vi "Dialog Box.vi"(8 "error in (no error)":errorcluster, 11 "Dialog in":refnum<class "Dialog.lvclass">) -> (0 "error out":errorcluster, 1 "timed out?":bool, 2 "Selection":string, 3 "Dialog out":refnum<class "Dialog.lvclass">)   [LabVIEW 2012, in "Dialog.lvlib" / "Dialog.lvclass"]
doc: "This VI contains the code for the dialog box.\nOverride this VI to provide more functionality or to create your own application-specific dialog box."
uses:
  Dialog.lvclass
  Fading/_Fade In(I32).vi
panel:
  out "String":string
  in  "OK Button":bool
  # "Message"
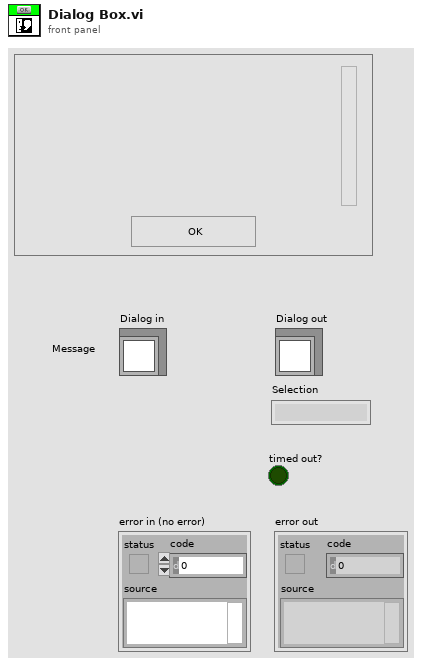
[diagram p1: front panel]
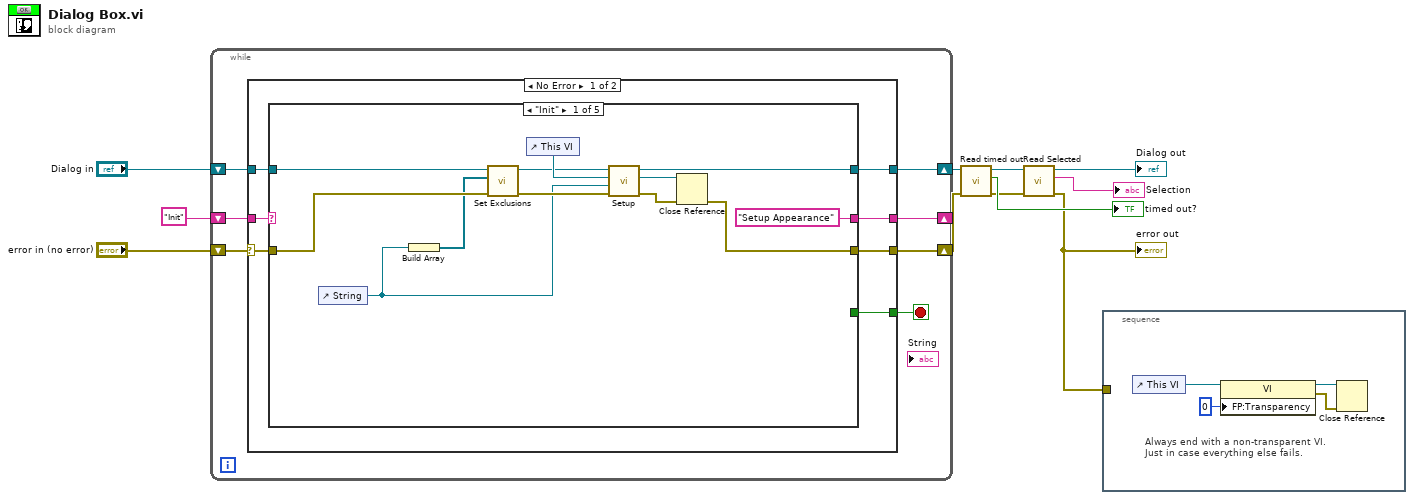
[diagram p0: block diagram]
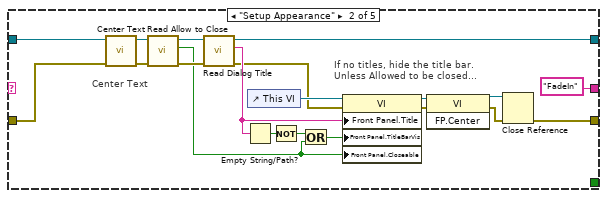
[diagram p2: hidden frame]
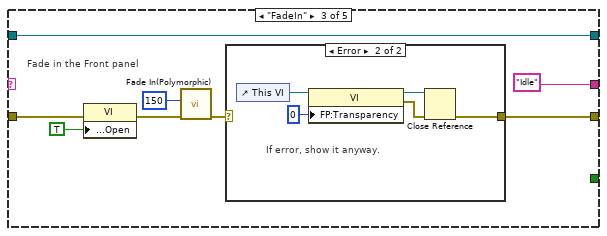
[diagram p3: hidden frame]
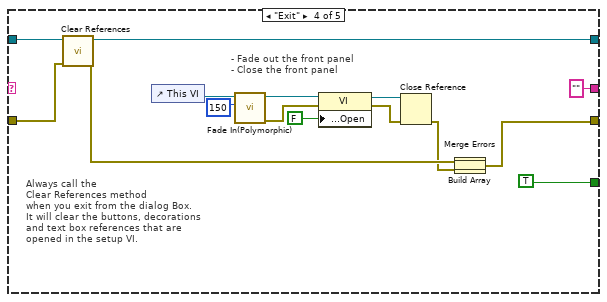
[diagram p5: hidden frame]
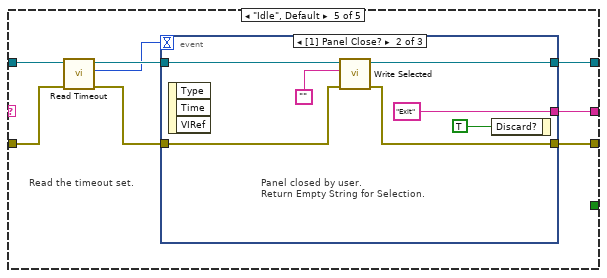
[diagram p6: hidden frame]
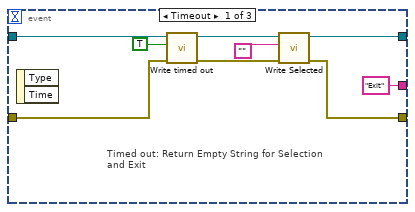
[diagram p7: hidden frame]
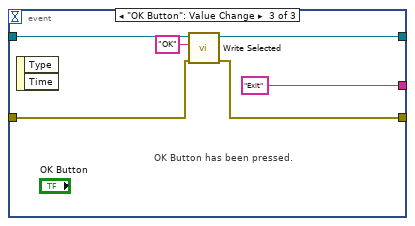
[diagram p8: hidden frame]
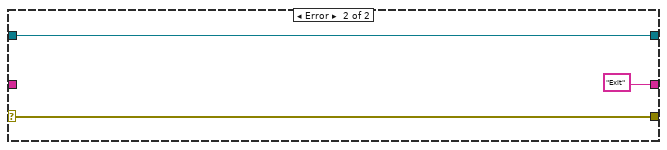
[diagram p9: hidden frame]
diagram:
  n1 = while {
    shift-right: [w14] -> _
    shift-left: "Init" -> [w15]
    shift-right: [w18] -> w4
    shift-left: "Dialog in" -> [w17]
    shift-right: [w16] -> w3
    shift-left: "error in (no error)" -> [w12]
    stop <- w13 stop-if-true
    n2 = case shown="No Error" w12 {
      selector: w12 -> [w19 w120]
      tunnel: [w25 w118] -> w18
      tunnel: w17 -> [w24 w118]
      tunnel: [w23 w120] -> w16
      tunnel: w15 -> [w22 _]
      tunnel: [w21 "Exit"] -> w14
      tunnel: [w20 _] -> w13
      frame No Error {
        n3 = case shown="\"Init\"" w22 {
          tunnel: [w35 w48 w65 w77 w95] -> w25
          tunnel: w24 -> [w31 w39 w65 w78 w92]
          tunnel: [w32 w49 w61 w73 w94] -> w23
          tunnel: w19 -> [w28 w38 w60 w76 w89]
          tunnel: ["Setup Appearance" "FadeIn" "Idle" "" w93] -> w21
          tunnel: [_ _ _ TRUE _] -> w20
          frame "Init" {
            n4 = control-ref of="String"() -> (w27:refnum<vi>)
            n5 = Build Array(w27) -> (w26:refnum<vi>[])
            n6 = call-dynamic "Set Exclusions.vi"("error in (no error)"=w28, "Exclusions"=w26, "Dialog in"=w31) -> ("error out"=w29:errorcluster, "Dialog out"=w30:refnum<class "Dialog.lvclass">)  [unwired: 7 out]
            n7 = control-ref of="This VI"() -> (w36:refnum<vi>)
            n8 = call-dynamic "Setup.vi"("error in (no error)"=w29, "Str Refnum"=w27, "VI Reference"=w36, "Dialog in"=w30) -> ("error out"=w33:errorcluster, "VI reference (dup)"=w34:refnum<vi>, "Dialog out"=w35:refnum<class "Dialog.lvclass">)  [unwired: 5 out]
            n9 = Close Reference(reference=w34, error in (no error)=w33) -> (error out=w32:errorcluster)
          }
          frame "Setup Appearance" {
            # "Center Text"
            # "If no titles, hide the title bar.\nUnless Allowed to be closed..."
            n10 = call-dynamic "Center Text.vi"("error in (no error)"=w38, "Dialog in"=w39) -> ("error out"=w44:errorcluster, "Dialog out"=w46:refnum<class "Dialog.lvclass">)  [unwired: 1 in, 7 out]
            n11 = call-dynamic "Read Allow to Close.vi"("error in (no error)"=w44, "Dialog.lvclass in"=w46) -> ("error out"=w43:errorcluster, "Allow to close?"=w40:bool, "Dialog.lvclass out"=w45:refnum<class "Dialog.lvclass">)  [unwired: 7 out]
            n12 = call-dynamic "Read Dialog Title.vi"("error in (no error)"=w43, "Dialog in"=w45) -> ("error out"=w47:errorcluster, "Dialog Title"=w52:string, "Dialog out"=w48:refnum<class "Dialog.lvclass">)  [unwired: 7 out]
            n13 = Empty String/Path?(string/path=w52) -> (empty?=w55:bool)
            n14 = control-ref of="This VI"() -> (w56:refnum<vi>)
            n15 = Not(x=w55) -> (.not. x?=w42:bool)
            n16 = Or(x=w42, y=w40) -> (x .or. y?=w41:bool)
            n17 = property class="VI"(reference=w56, error in=w47, "Front Panel.Title"=w52, "Front Panel.TitleBarVis"=w41, "Front Panel.Closeable"=w40) -> (reference out=w54:refnum<vi>, error out=w53:errorcluster)
            n18 = invoke class="VI" method="FP.Center"(reference=w54, error in=w53) -> (reference out=w51:refnum<vi>, error out=w50:errorcluster)  [unwired: 1 in, 1 out]
            n19 = Close Reference(reference=w51, error in (no error)=w50) -> (error out=w49:errorcluster)
          }
          frame "FadeIn" {
            # "Fade in the Front panel"
            n20 = property class="VI"(error in=w60, "Front Panel.Open"=TRUE ("Front Panel Window:Open")) -> (error out=w59:errorcluster)  [unwired: 1 in, 1 out]
            n21 = call-poly "Fade In(Polymorphic).vi"("error in"=w59, "Fade time (ms)"=150) -> ("error out"=w62:errorcluster)  [unwired: 2 in, 7 out]
            n22 = case shown="Error" w62 {
              selector: w62 -> [w66 _]
              tunnel: [w66 w67] -> w61
              frame No Error {
              }
              frame Error {
                # "If error, show it anyway."
                n23 = control-ref of="This VI"() -> (w69:refnum<vi>)
                n24 = property class="VI"(reference=w69, "FP:Transparency"=u8 0 ("Front Panel Window:Transparency")) -> (reference out=w70:refnum<vi>, error out=w71:errorcluster)  [unwired: 1 in]
                n25 = Close Reference(reference=w70, error in (no error)=w71) -> (error out=w67:errorcluster)
              }
            }
          }
          frame "Exit" {
            # "Always call the\nClear References method\nwhen you exit from the dialog Box.\nIt will clear the buttons, decorations\nand text box references that are \nopened in the setup VI."
            # "- Fade out the front panel\n- Close the front panel"
            n26 = call-dynamic "Clear References.vi"("error in (no error)"=w76, "Dialog in"=w78) -> ("error out"=w75:errorcluster, "Dialog out"=w77:refnum<class "Dialog.lvclass">)  [unwired: 8 out]
            n27 = control-ref of="This VI"() -> (w84:refnum<vi>)
            n28 = call-poly "Fade In(Polymorphic).vi"("Fade time (ms)"=150, "VI Reference (calling VI)"=w84) -> ("error out"=w82:errorcluster, "dup VI Reference"=w83:refnum<vi>)  [unwired: 2 in, 6 out]
            n29 = property class="VI"(reference=w83, error in=w82, "Front Panel.Open"=FALSE ("Front Panel Window:Open")) -> (reference out=w80:refnum<vi>, error out=w79:errorcluster)
            n30 = Close Reference(reference=w80, error in (no error)=w79) -> (error out=w74:errorcluster)
            n31 = Build Array(w75, w74) -> (w72:errorcluster[])
            n32 = Merge Errors(w72) -> (w73:errorcluster)
          }
          frame "Idle", Default {
            # "Read the timeout set."
            n33 = call-dynamic "Read Timeout.vi"("error in (no error)"=w89, "Dialog.lvclass in"=w92) -> ("error out"=w88:errorcluster, "Timeout"=w90:i32, "Dialog.lvclass out"=w91:refnum<class "Dialog.lvclass">)  [unwired: 7 out]
            n34 = event shown="[1] Panel Close?" {
              selector: _ -> [_ _ _]
              dyn-events: _ -> [_ _ _]
              timeout: w90 -> [_ _ _]
              tunnel: [w97 w107 w115] -> w95
              tunnel: w91 -> [w103 w108 w116]
              tunnel: [w98 w105 w112] -> w94
              tunnel: w88 -> [w101 w106 w113]
              tunnel: ["Exit" "Exit" "Exit"] -> w93
              event Timeout {
                # "Timed out: Return Empty String for Selection\nand Exit"
                n35 = event-data() -> ()  [unwired: 3 out]
                n36 = call-dynamic "Write timed out.vi"("error in (no error)"=w101, "timed out?"=TRUE, "Dialog.lvclass in"=w103) -> ("error out"=w99:errorcluster, "Dialog.lvclass out"=w100:refnum<class "Dialog.lvclass">)  [unwired: 7 out]
                n37 = call-dynamic "Write Selected.vi"("error in (no error)"=w99, "Selected"="", "Dialog.lvclass in"=w100) -> ("error out"=w98:errorcluster, "Dialog.lvclass out"=w97:refnum<class "Dialog.lvclass">)  [unwired: 7 out]
              }
              event Panel Close? {
                # "Panel closed by user.\nReturn Empty String for Selection."
                n38 = event-data() -> ()  [unwired: 4 out]
                n39 = call-dynamic "Write Selected.vi"("error in (no error)"=w106, "Selected"="", "Dialog.lvclass in"=w108) -> ("error out"=w105:errorcluster, "Dialog.lvclass out"=w107:refnum<class "Dialog.lvclass">)  [unwired: 7 out]
                n40 = event-data("Discard?"=TRUE) -> ()  [unwired: 1 in, 1 out]
              }
              event "OK Button": Value Change {
                # "OK Button has been pressed."
                n41 = event-data() -> ()  [unwired: 3 out]
                n42 = call-dynamic "Write Selected.vi"("error in (no error)"=w113, "Selected"="OK", "Dialog.lvclass in"=w116) -> ("error out"=w112:errorcluster, "Dialog.lvclass out"=w115:refnum<class "Dialog.lvclass">)  [unwired: 7 out]
              }
            }
          }
        }
      }
      frame Error {
      }
    }
  }
  n43 = call-dynamic "Read timed out.vi"("error in (no error)"=w3, "Dialog.lvclass in"=w4) -> ("error out"=w1:errorcluster, "timed out?"=→"timed out?":bool, "Dialog.lvclass out"=w2:refnum<class "Dialog.lvclass">)  [unwired: 7 out]
  n44 = call-dynamic "Read Selected.vi"("error in (no error)"=w1, "Dialog.lvclass in"=w2) -> ("error out"=w6:errorcluster, "Selected"=→"Selection":string, "Dialog.lvclass out"=→"Dialog out":refnum<class "Dialog.lvclass">)  [unwired: 7 out]
  "error out" <- w6
  n45 = stacked-sequence {
    tunnel: w6 -> [_]
    frame #0 {
      # "Always end with a non-transparent VI.\nJust in case everything else fails."
      n46 = control-ref of="This VI"() -> (w123:refnum<vi>)
      n47 = property class="VI"(reference=w123, "FP:Transparency"=u8 0 ("Front Panel Window:Transparency")) -> (reference out=w122:refnum<vi>, error out=w121:errorcluster)  [unwired: 1 in]
      n48 = Close Reference(reference=w122, error in (no error)=w121) -> ()  [unwired: 1 out]
    }
  }
